vi "SetElectricDarkSample.vi"() -> ()   [LabVIEW 2012]
panel:
  in  "Enable Correct \nfor Electrical Dark":bool
  out "Spectrum of the first Spectrometer":cluster{"Y":dbl[], "Y":dbl[]}[](graph)
  in  "stop":bool
  in  "Enter the \nInetegration Time":i32
  in  "Start":bool=TRUE
  out "Number of Spectrometers":i32
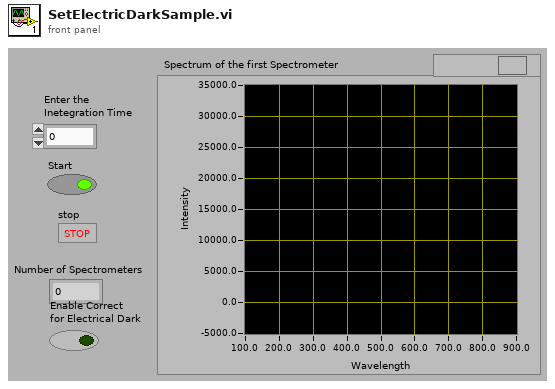
[diagram p1: front panel]
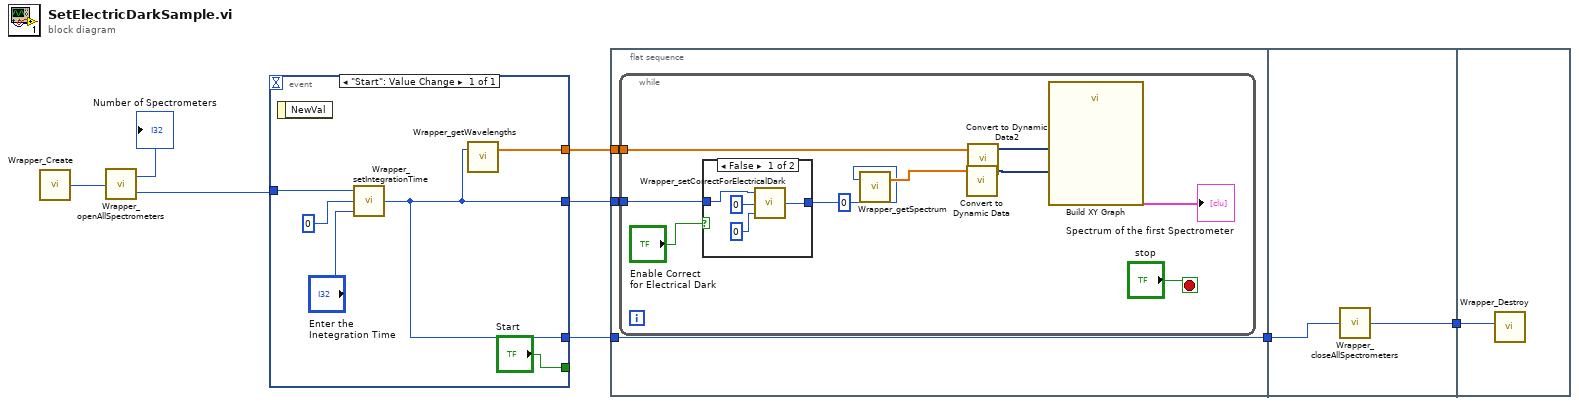
[diagram p0: block diagram]
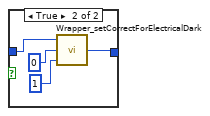
[diagram p2: hidden frame]
diagram:
  n1 = call <instrlib>:"Wrapper_Create.vi"() -> ("Wrapper"=w8:u64)
  n2 = call <instrlib>:"Wrapper_openAllSpectrometers.vi"("Wrapper In"=w8) -> ("Number of Spectrometers"=→"Number of Spectrometers":i32, "Wrapper Out"=w6:u64)
  n3 = event shown="[0] \"Start\": Value Change" {
    selector: _ -> [_]
    dyn-events: _ -> [_]
    timeout: _ -> [_]
    tunnel: ["Start"] -> _
    tunnel: w6 -> [w11]
    tunnel: [w9] -> w5
    tunnel: [w10] -> w4
    tunnel: [w9] -> w2
    event "Start": Value Change {
      n4 = event-data() -> ()  [unwired: 1 in, 1 out]
      n5 = call <instrlib>:"Wrapper_setIntegrationTime.vi"("Integration Time"="Enter the \nInetegration Time", "Index"=0, "Wrapper In"=w11) -> ("Wrapper Out"=w9:u64)
      n6 = call <instrlib>:"Wrapper_getWavelengths.vi"("Wrapper"=w9) -> ("WL Values"=w10:dbl[])  [unwired: 1 in, 1 out]
    }
  }
  n7 = flat-sequence {
    tunnel: w5 -> [w17]
    tunnel: w4 -> [w16]
    tunnel: [w15] -> w3
    tunnel: w2 -> [w15]
    tunnel: w3 -> [w37]
    tunnel: [w36] -> w1
    tunnel: w1 -> [w38]
    frame #0 {
      n8 = while {
        tunnel: w17 -> [w19]
        tunnel: w16 -> [w22]
        stop <- "stop" stop-if-true
        n9 = case shown="False" "Enable Correct \nfor Electrical Dark" {
          tunnel: w19 -> [w30 w34]
          tunnel: [w31 w35] -> w18
          frame False {
            n10 = call <instrlib>:"Wrapper_setCorrectForElectricalDark.vi"("On/Off"=0, "Index"=0, "Wrapper In"=w30) -> ("Wrapper Out"=w31:u64)
          }
          frame True {
            n11 = call <instrlib>:"Wrapper_setCorrectForElectricalDark.vi"("On/Off"=1, "Index"=0, "Wrapper In"=w34) -> ("Wrapper Out"=w35:u64)
          }
        }
        n12 = call <instrlib>:"Wrapper_getSpectrum.vi"("Index"=0, "Wrapper"=w18) -> ("Spectrum Values"=w24:dbl[])  [unwired: 1 out]
        n13 = call "Convert to Dynamic Data"("Array"=w24) -> ("Dynamic Data Type"=w23:dynamicdata)  [unwired: 3 in]
        n14 = call "Convert to Dynamic Data2"("Array"=w22) -> ("Dynamic Data Type"=w21:dynamicdata)  [unwired: 3 in]
        n15 = call "Build XY Graph"("Y Input"=w23, "X Input"=w21) -> ("XY Graph"=→"Spectrum of the first Spectrometer":cluster{"Y":dbl[], "Y":dbl[]}[])  [unwired: 8 in, 1 out]
      }
    }
    frame #1 {
      n16 = call <instrlib>:"Wrapper_closeAllSpectrometers.vi"("Wrapper In"=w37) -> ("Wrapper Out"=w36:u64)
    }
    frame #2 {
      n17 = call <instrlib>:"Wrapper_Destroy.vi"("Wrapper"=w38) -> ()
    }
  }
